vi "ArduinoRead.vi"(6 "Command String":string, 7 "Arduino function":T1(ring), 8 "error in (no error)":errorcluster, 9 "Humidity IN":dbl[](array[numeric]), 10 "Temperature IN":dbl[](array[numeric]), 11 "ArduinoControl in":refnum<class "ArduinoControl.lvclass">) -> (0 "error out":errorcluster, 1 "rel. Humidity [%]":dbl, 2 "Temperature [°C]":dbl, 3 "ArduinoControl out":refnum<class "ArduinoControl.lvclass">, 4 "Interlock Status":u16(ring) items=["Dark", "Light"], 5 "Edgesense Status":u16(ring)=1 items=["Contact", "No contact"])   [LabVIEW 2018, in "ArduinoControl.lvclass"]
uses:
  ArduinoControl.lvclass
  ArduinoControl.lvclass/ArduinoControl.ctl
panel:
  out "return count 2":u32
  out "Humidity OUT":dbl[](array[numeric])
  out "Temperature OUT":dbl[](array[numeric])
  out "return count":u32
  out "String":string
  out "VISA resource name OUT":refnum<visa-resource-name>="COM24"
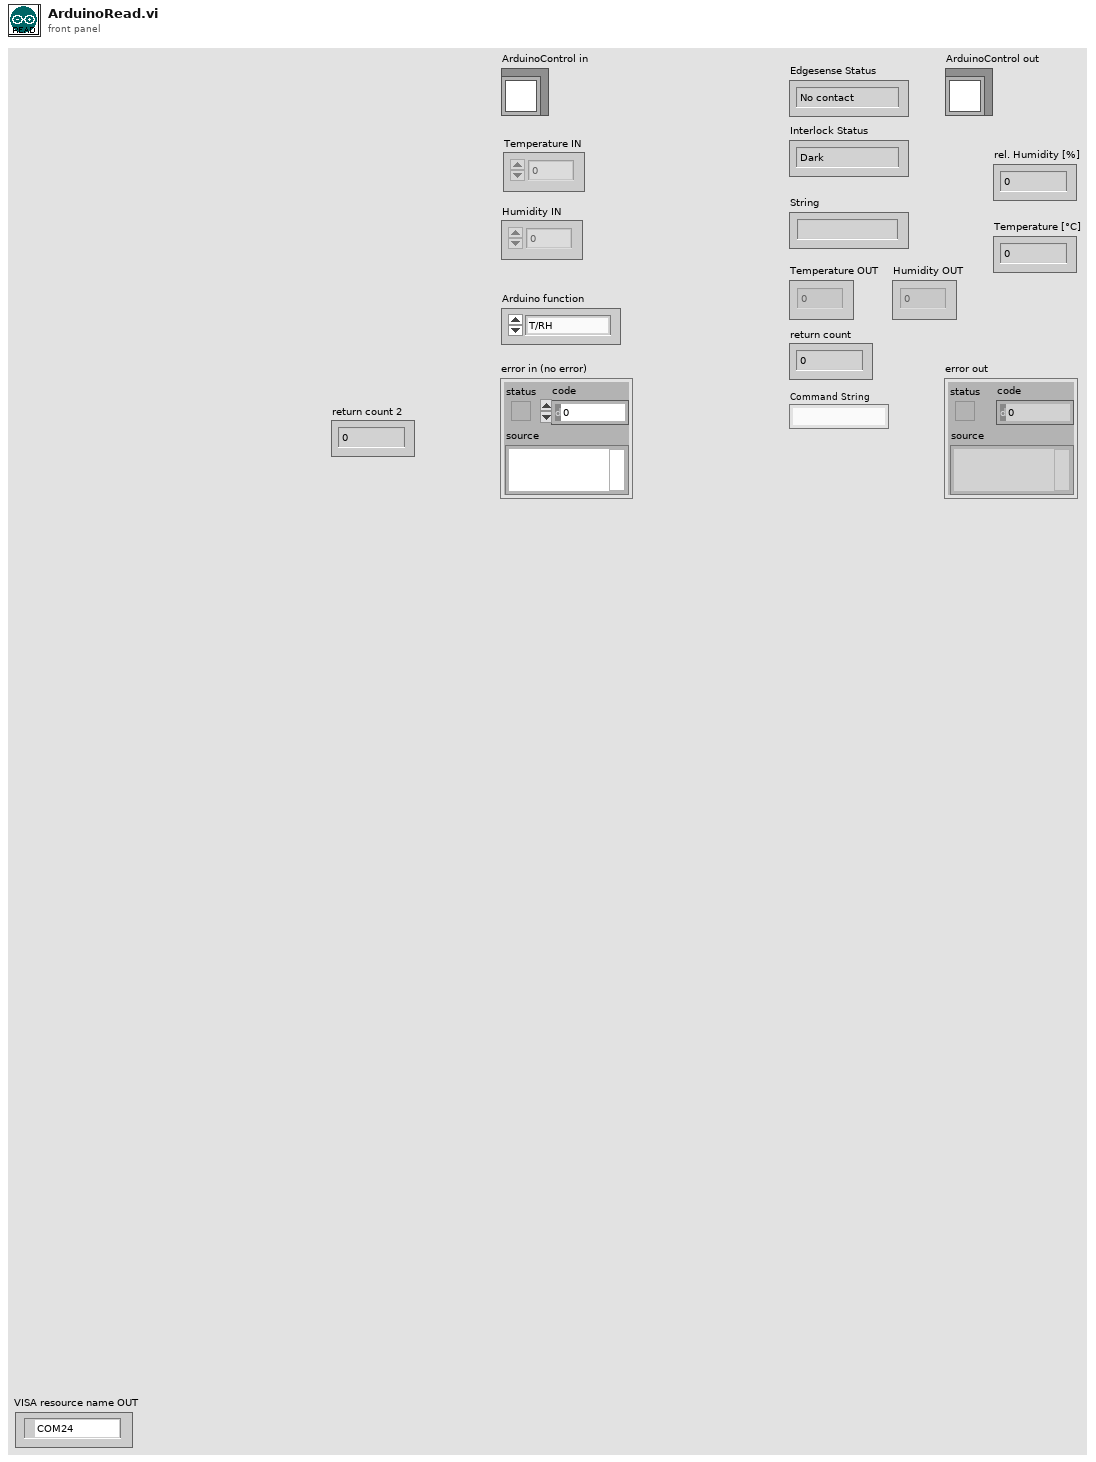
[diagram p1: front panel]
types:
  T1 = enum16{"T/RH", "Interlock", "Edgesense", "Open Switch", "Close Switch", "Reset Switches"}
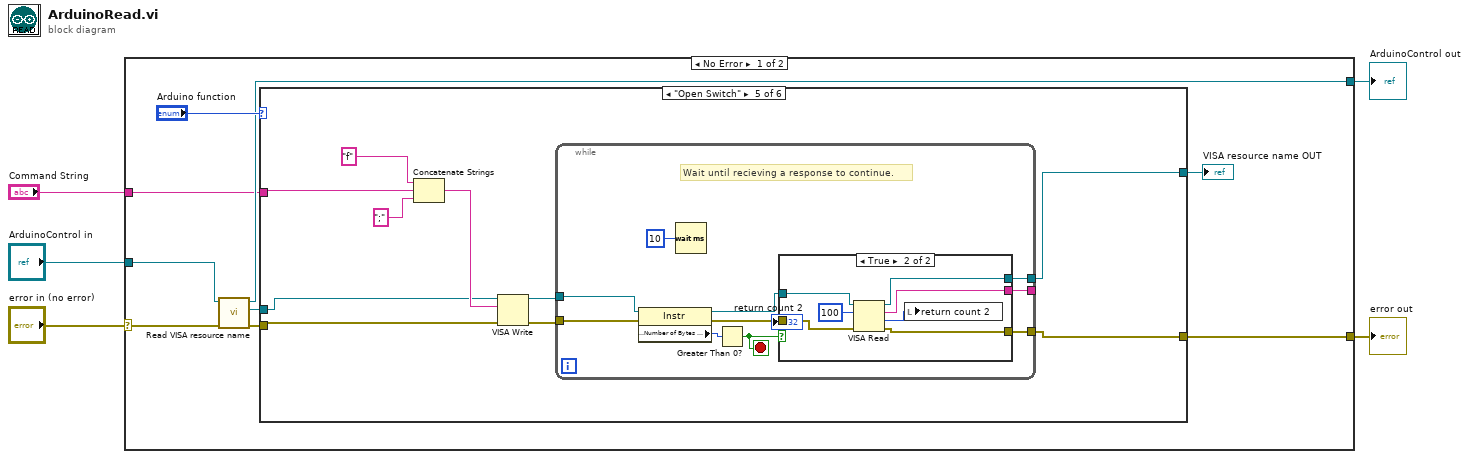
[diagram p0: block diagram]
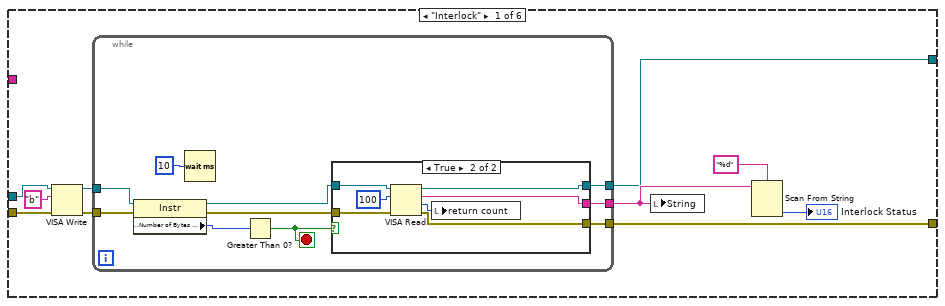
[diagram p2: hidden frame]
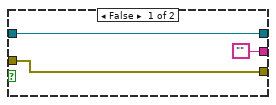
[diagram p3: hidden frame]
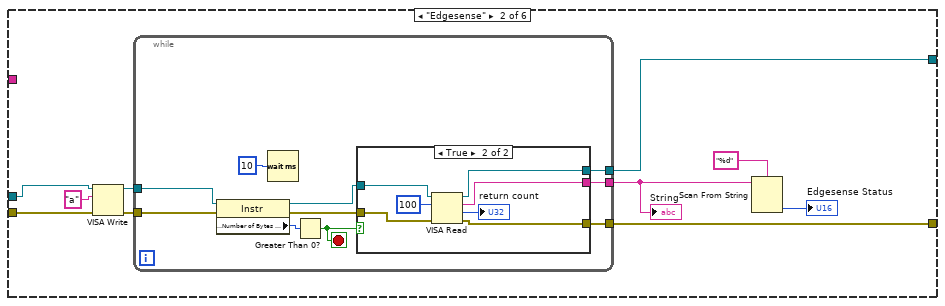
[diagram p4: hidden frame]
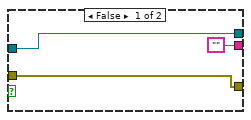
[diagram p5: hidden frame]
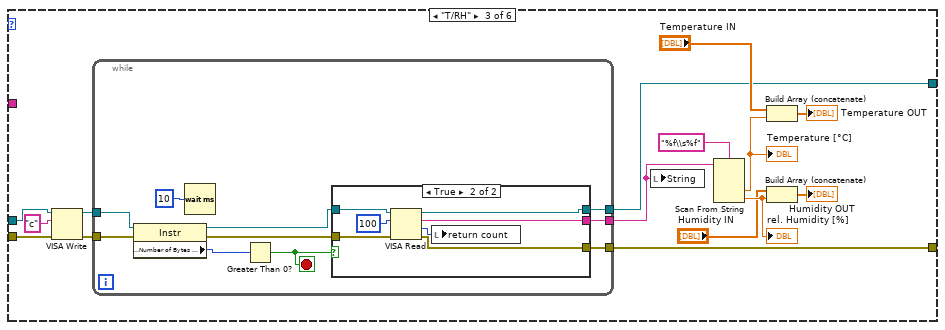
[diagram p6: hidden frame]
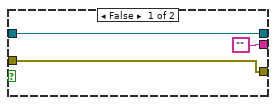
[diagram p7: hidden frame]
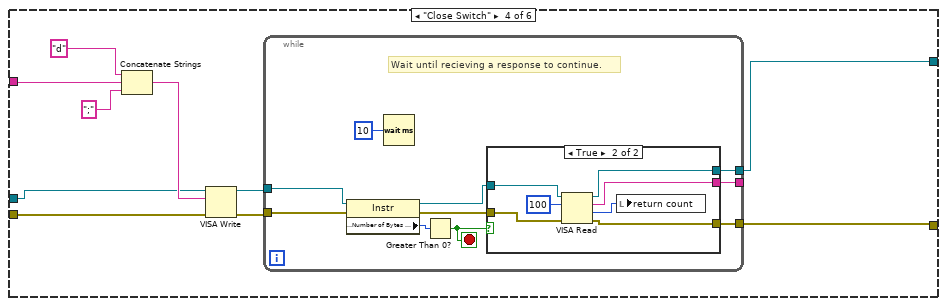
[diagram p8: hidden frame]
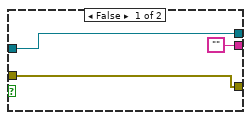
[diagram p9: hidden frame]
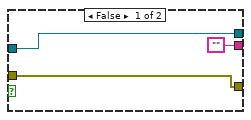
[diagram p10: hidden frame]
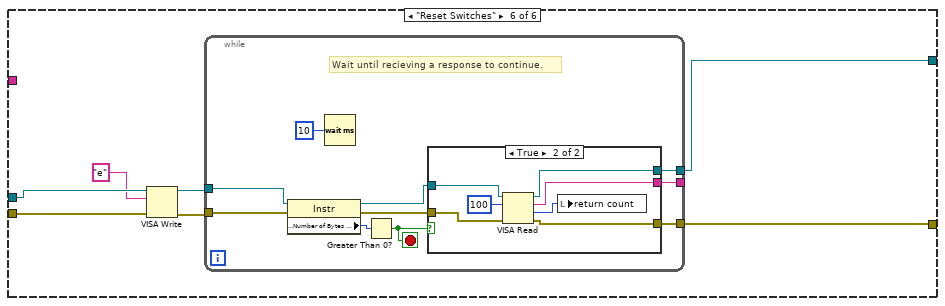
[diagram p11: hidden frame]
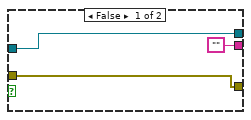
[diagram p12: hidden frame]
diagram:
  n1 = case shown="No Error" "error in (no error)" {
    selector: "error in (no error)" -> [w9 w198]
    tunnel: [w10 w197] -> w3
    tunnel: "ArduinoControl in" -> [w11 w197]
    tunnel: [w12 w198] -> w2
    tunnel: "Command String" -> [w6 _]
    frame No Error {
      n2 = call "Read VISA resource name.vi"("error in (no error)"=w9, "ArduinoControl in"=w11) -> ("error out"=w8:errorcluster, "VISA resource name"=w7:refnum<visa-resource-name>, "ArduinoControl out"=w10:refnum<class "ArduinoControl.lvclass">)  [unwired: 7 in]
      n3 = case shown="\"Open Switch\"" "Arduino function" {
        tunnel: w8 -> [w16 w47 w77 w119 w141 w173]
        tunnel: w7 -> [w18 w48 w79 w114 w142 w174]
        tunnel: [w21 w50 w80 w111 w144 w171] -> w13
        tunnel: [w20 w51 w81 w110 w140 w170] -> w12
        tunnel: w6 -> [_ _ _ w117 w143 _]
        frame "Interlock" {
          n4 = VISA Write(VISA resource name=w18, write buffer="b", error in (no error)=w16) -> (VISA resource name out=w17:refnum<visa-resource-name>, error out=w15:errorcluster)  [unwired: 1 out]
          n5 = while {
            tunnel: [w32] -> w21
            tunnel: [w31] -> w22
            tunnel: w15 -> [w25]
            tunnel: w17 -> [w26]
            tunnel: [w30] -> w20
            stop <- w27 stop-if-true
            n6 = property class="Instr"(reference=w26, error in=w25) -> (reference out=w34:refnum<visa-resource-name>, error out=w33:errorcluster, "Serial Settings:Number of Bytes at Serial Port"=w28:u32)
            n7 = Wait (ms)(milliseconds to wait=10) -> ()  [unwired: 1 out]
            n8 = Greater Than 0?(x=w28) -> (x > 0?=w27:bool)
            n9 = case shown="True" w27 {
              tunnel: w34 -> [w35 w44]
              tunnel: w33 -> [w36 w43]
              tunnel: [w35 w42] -> w32
              tunnel: ["" w41] -> w31
              tunnel: [w36 w40] -> w30
              frame False {
              }
              frame True {
                n10 = VISA Read(VISA resource name=w44, byte count=100, error in (no error)=w43) -> (VISA resource name out=w42:refnum<visa-resource-name>, read buffer=w41:string, return count=w39:u32, error out=w40:errorcluster)
                n11 = local write "return count"(w39) -> ()
              }
            }
          }
          n12 = local write "String"(w22) -> ()
          n13 = Scan From String(format string="%d", input string=w22) -> (output 1=→"Interlock Status":u16)  [unwired: 3 in, 3 out]
        }
        frame "Edgesense" {
          n14 = VISA Write(VISA resource name=w48, write buffer="a", error in (no error)=w47) -> (VISA resource name out=w46:refnum<visa-resource-name>, error out=w45:errorcluster)  [unwired: 1 out]
          n15 = while {
            tunnel: [w62] -> w50
            tunnel: [w61] -> w52
            tunnel: w46 -> [w57]
            tunnel: [w60] -> w51
            tunnel: w45 -> [w58]
            stop <- w55 stop-if-true
            n16 = property class="Instr"(reference=w57, error in=w58) -> (reference out=w64:refnum<visa-resource-name>, error out=w63:errorcluster, "Serial Settings:Number of Bytes at Serial Port"=w56:u32)
            n17 = Wait (ms)(milliseconds to wait=10) -> ()  [unwired: 1 out]
            n18 = Greater Than 0?(x=w56) -> (x > 0?=w55:bool)
            n19 = case shown="True" w55 {
              tunnel: w64 -> [w65 w74]
              tunnel: w63 -> [w66 w73]
              tunnel: [w65 w72] -> w62
              tunnel: ["" w71] -> w61
              tunnel: [w66 w70] -> w60
              frame False {
              }
              frame True {
                n20 = VISA Read(VISA resource name=w74, byte count=100, error in (no error)=w73) -> (VISA resource name out=w72:refnum<visa-resource-name>, read buffer=w71:string, return count=→"return count":u32, error out=w70:errorcluster)
              }
            }
          }
          "String" <- w52
          n21 = Scan From String(format string="%d", input string=w52) -> (output 1=→"Edgesense Status":u16)  [unwired: 3 in, 3 out]
        }
        frame "T/RH" {
          n22 = VISA Write(VISA resource name=w79, write buffer="c", error in (no error)=w77) -> (VISA resource name out=w75:refnum<visa-resource-name>, error out=w76:errorcluster)  [unwired: 1 out]
          n23 = while {
            tunnel: [w97] -> w80
            tunnel: [w96] -> w82
            tunnel: w76 -> [w91]
            tunnel: w75 -> [w90]
            tunnel: [w95] -> w81
            stop <- w92 stop-if-true
            n24 = property class="Instr"(reference=w90, error in=w91) -> (reference out=w99:refnum<visa-resource-name>, error out=w98:errorcluster, "Serial Settings:Number of Bytes at Serial Port"=w93:u32)
            n25 = Wait (ms)(milliseconds to wait=10) -> ()  [unwired: 1 out]
            n26 = Greater Than 0?(x=w93) -> (x > 0?=w92:bool)
            n27 = case shown="True" w92 {
              tunnel: w99 -> [w100 w109]
              tunnel: w98 -> [w101 w108]
              tunnel: [w100 w107] -> w97
              tunnel: ["" w106] -> w96
              tunnel: [w101 w105] -> w95
              frame False {
              }
              frame True {
                n28 = VISA Read(VISA resource name=w109, byte count=100, error in (no error)=w108) -> (VISA resource name out=w107:refnum<visa-resource-name>, read buffer=w106:string, return count=w103:u32, error out=w105:errorcluster)
                n29 = local write "return count"(w103) -> ()
              }
            }
          }
          n30 = local write "String"(w82) -> ()
          n31 = Scan From String(format string="%f\\s%f", input string=w82) -> (output 1=w84:dbl, output 2=w89:dbl)  [unwired: 4 in, 3 out]
          "rel. Humidity [%]" <- w89
          "Temperature [°C]" <- w84
          n32 = Build Array (concatenate)("Temperature IN", w84) -> (→"Temperature OUT":dbl[])
          n33 = Build Array (concatenate)("Humidity IN", w89) -> (→"Humidity OUT":dbl[])
        }
        frame "Close Switch" {
          n34 = Concatenate Strings("d", w117, ";" ("string")) -> (w115:string)
          n35 = VISA Write(VISA resource name=w114, write buffer=w115, error in (no error)=w119) -> (VISA resource name out=w113:refnum<visa-resource-name>, error out=w112:errorcluster)  [unwired: 1 out]
          n36 = while {
            tunnel: [w127] -> w111
            tunnel: [w126] -> _
            tunnel: w113 -> [w122]
            tunnel: [w125] -> w110
            tunnel: w112 -> [w123]
            stop <- w120 stop-if-true
            # "Wait until recieving a response to continue."
            n37 = property class="Instr"(reference=w122, error in=w123) -> (reference out=w129:refnum<visa-resource-name>, error out=w128:errorcluster, "Serial Settings:Number of Bytes at Serial Port"=w121:u32)
            n38 = Wait (ms)(milliseconds to wait=10) -> ()  [unwired: 1 out]
            n39 = Greater Than 0?(x=w121) -> (x > 0?=w120:bool)
            n40 = case shown="True" w120 {
              tunnel: w129 -> [w130 w139]
              tunnel: w128 -> [w131 w138]
              tunnel: [w130 w137] -> w127
              tunnel: ["" w136] -> w126
              tunnel: [w131 w135] -> w125
              frame False {
              }
              frame True {
                n41 = VISA Read(VISA resource name=w139, byte count=100, error in (no error)=w138) -> (VISA resource name out=w137:refnum<visa-resource-name>, read buffer=w136:string, return count=w133:u32, error out=w135:errorcluster)
                n42 = local write "return count"(w133) -> ()
              }
            }
          }
        }
        frame "Open Switch" {
          n43 = Concatenate Strings("f", w143, ";" ("string")) -> (w147:string)
          n44 = VISA Write(VISA resource name=w142, write buffer=w147, error in (no error)=w141) -> (VISA resource name out=w146:refnum<visa-resource-name>, error out=w145:errorcluster)  [unwired: 1 out]
          n45 = while {
            tunnel: [w157] -> w144
            tunnel: [w156] -> _
            tunnel: w146 -> [w152]
            tunnel: [w155] -> w140
            tunnel: w145 -> [w153]
            stop <- w150 stop-if-true
            # "Wait until recieving a response to continue."
            n46 = property class="Instr"(reference=w152, error in=w153) -> (reference out=w159:refnum<visa-resource-name>, error out=w158:errorcluster, "Serial Settings:Number of Bytes at Serial Port"=w151:u32)
            n47 = Wait (ms)(milliseconds to wait=10) -> ()  [unwired: 1 out]
            n48 = Greater Than 0?(x=w151) -> (x > 0?=w150:bool)
            n49 = case shown="True" w150 {
              tunnel: w159 -> [w160 w169]
              tunnel: w158 -> [w161 w168]
              tunnel: [w160 w167] -> w157
              tunnel: ["" w166] -> w156
              tunnel: [w161 w165] -> w155
              frame False {
              }
              frame True {
                n50 = VISA Read(VISA resource name=w169, byte count=100, error in (no error)=w168) -> (VISA resource name out=w167:refnum<visa-resource-name>, read buffer=w166:string, return count=w163:u32, error out=w165:errorcluster)
                n51 = local write "return count 2"(w163) -> ()
              }
            }
          }
        }
        frame "Reset Switches" {
          n52 = VISA Write(VISA resource name=w174, write buffer="e", error in (no error)=w173) -> (VISA resource name out=w176:refnum<visa-resource-name>, error out=w175:errorcluster)  [unwired: 1 out]
          n53 = while {
            tunnel: [w184] -> w171
            tunnel: [w183] -> _
            tunnel: w176 -> [w179]
            tunnel: [w182] -> w170
            tunnel: w175 -> [w180]
            stop <- w177 stop-if-true
            # "Wait until recieving a response to continue."
            n54 = property class="Instr"(reference=w179, error in=w180) -> (reference out=w186:refnum<visa-resource-name>, error out=w185:errorcluster, "Serial Settings:Number of Bytes at Serial Port"=w178:u32)
            n55 = Wait (ms)(milliseconds to wait=10) -> ()  [unwired: 1 out]
            n56 = Greater Than 0?(x=w178) -> (x > 0?=w177:bool)
            n57 = case shown="True" w177 {
              tunnel: w186 -> [w187 w196]
              tunnel: w185 -> [w188 w195]
              tunnel: [w187 w194] -> w184
              tunnel: ["" w193] -> w183
              tunnel: [w188 w192] -> w182
              frame False {
              }
              frame True {
                n58 = VISA Read(VISA resource name=w196, byte count=100, error in (no error)=w195) -> (VISA resource name out=w194:refnum<visa-resource-name>, read buffer=w193:string, return count=w190:u32, error out=w192:errorcluster)
                n59 = local write "return count"(w190) -> ()
              }
            }
          }
        }
      }
      "VISA resource name OUT" <- w13
    }
    frame Error {
    }
  }
  "error out" <- w2
  "ArduinoControl out" <- w3
